vi "5060_check_outputs.vi"(1 "Address (Main, Sub reqd.)":T1, 2 "Channel Name":string) -> (3 "Comment":string, 4 "All chs.":u8 format="%.0b", 5 "Single Channel":i16)   [LabVIEW 2018]
uses:
  ADAM Client/Sub VIs/ADAM Controls/Address.ctl
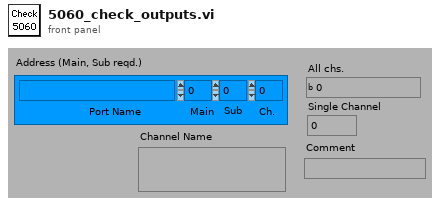
[diagram p1: front panel]
types:
  T1 = typedef "Address.ctl" = cluster{"Main":i32, "Ch.":i32, "Sub":i32, "Port Name":string}
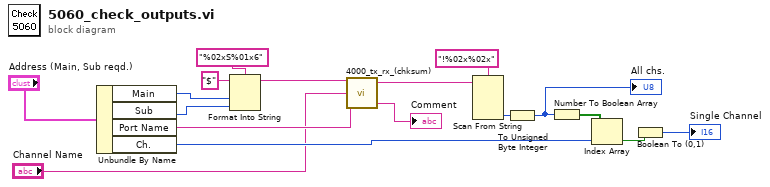
[diagram p0: block diagram]
diagram:
  n1 = Unbundle By Name("Address (Main, Sub reqd.)") -> ("Main"=w16:i32, "Sub"=w17:i32, "Port Name"=w9:string, "Ch."=w6:i32)
  n2 = Format Into String(format string="%02xS%01x6", initial string="$", w16, w17) -> (resulting string=w13:string)  [unwired: 1 in, 1 out]
  n3 = call "4000_tx_rx_(chksum).vi"("Write String"=w13, "Channel Name"="Channel Name", "Port Name"=w9) -> ("Read"=w8:string, "Comment out"=→"Comment":string)  [unwired: 2 in, 1 out]
  n4 = Scan From String(format string="!%02x%02x", input string=w8) -> (output 2=w7:u32)  [unwired: 2 in, 6 out]
  n5 = To Unsigned Byte Integer(number=w7) -> (unsigned 8bit integer=w5:u8)
  "All chs." <- w5
  n6 = Number To Boolean Array(number=w5) -> (Boolean array=w4:bool[])
  n7 = Index Array(array=w4, index=w6) -> (element=w3:bool)
  n8 = Boolean To (0,1)(Boolean=w3) -> (0, 1=→"Single Channel":i16)
